vi "Core Handle Error.vi"(8 "error in (no error)":errorcluster, 11 "CIFTemplateNode in":refnum<class "CIFCorePlugin.lvclass">) -> (0 "error out":errorcluster, 3 "CIFTemplateNode out":refnum<class "CIFCorePlugin.lvclass">)   [LabVIEW 2021, in "CIFCorePlugin.lvclass"]
uses:
  CIFCorePlugin.lvclass
  CIFCorePlugin.lvclass/CIFCorePlugin.ctl
  Typedef/Energized States.ctl
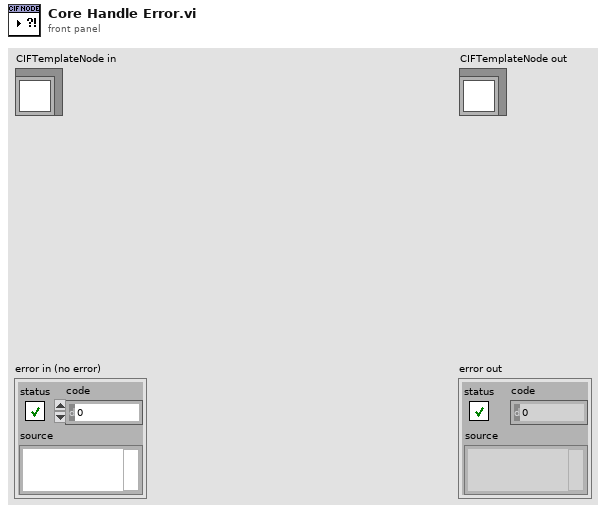
[diagram p1: front panel]
types:
  T1 = typedef "CIFCorePlugin.lvclass/Energized States.ctl" = enum16{"Prepare", "Execute", "Destroy"}
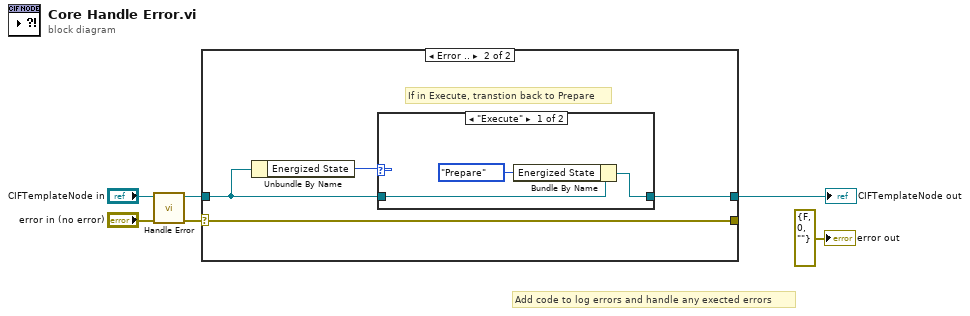
[diagram p0: block diagram]
diagram:
  # "Add code to log errors and handle any exected errors"
  n1 = call-dynamic "Handle Error.vi"("error in (no error)"="error in (no error)", "CIFTemplateNode in"="CIFTemplateNode in") -> ("error out"=w1:errorcluster, "CIFTemplateNode out"=w3:refnum<class "CIFCorePlugin.lvclass">)  [unwired: 8 in]
  n2 = case shown="Error .." w1 {
    selector: w1 -> [w7 w9]
    tunnel: [w8 w11] -> w6
    tunnel: w3 -> [w8 w10]
    tunnel: [w7 w9] -> _
    frame No Error {
    }
    frame Error {
      # "If in Execute, transtion back to Prepare"
      n3 = Unbundle By Name(w10) -> ("Energized State"=w12:T1)
      n4 = case shown="\"Execute\"" w12 {
        tunnel: [w14 w16] -> w11
        tunnel: w10 -> [w15 w16]
        frame "Execute" {
          n5 = Bundle By Name(cluster=w15, "Energized State"=Energized_States."Prepare") -> (w14:refnum<class "CIFCorePlugin.lvclass">)
        }
        frame "Destroy", Default {
        }
      }
    }
  }
  "CIFTemplateNode out" <- w6
  "error out" <- errorcluster {"status"=FALSE, "code"=0, "source"=""} ("error out")
